vi "Inj_Array_Split.vi"(10 "Inject_Arrays":dbl[](array[numeric]), 11 "Omicron":bool) -> (0 "Air Add":dbl[](array[numeric]), 1 "Air Cyc":dbl[](array[numeric]), 2 "HC Add":dbl[](array[numeric]), 3 "HC Cyc":dbl[](array[numeric]), 4 "O2":dbl[](array[numeric]), 5 "CO":dbl[](array[numeric]), 6 "NO":dbl[](array[numeric]), 9 "Cycle Length":i32)   [LabVIEW 2014]
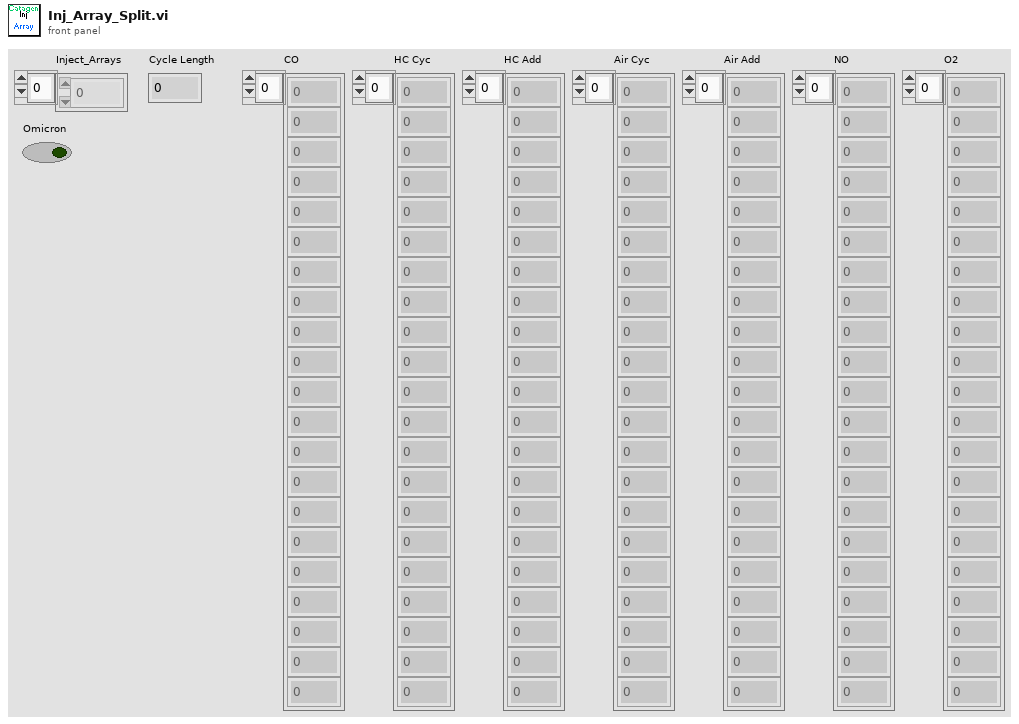
[diagram p1: front panel]
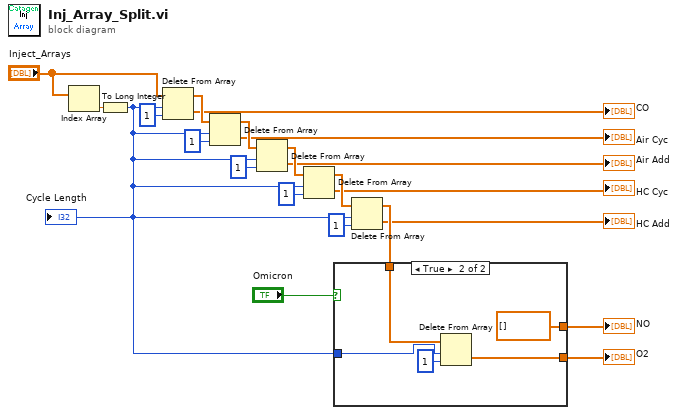
[diagram p0: block diagram]
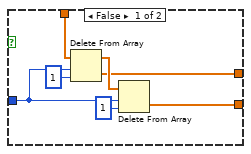
[diagram p2: hidden frame]
diagram:
  n1 = Index Array(array="Inject_Arrays") -> (element=w20:dbl)  [unwired: 1 in]
  n2 = To Long Integer(number=w20) -> (32bit integer=w2:i32)
  "Cycle Length" <- w2
  n3 = Delete From Array(array="Inject_Arrays", length=w2, index=1) -> (deleted portion=→"CO":dbl[], array with subset deleted=w19:dbl[])
  n4 = Delete From Array(array=w19, length=w2, index=1) -> (deleted portion=→"Air Cyc":dbl[], array with subset deleted=w18:dbl[])
  n5 = Delete From Array(array=w18, length=w2, index=1) -> (deleted portion=→"Air Add":dbl[], array with subset deleted=w15:dbl[])
  n6 = Delete From Array(array=w15, length=w2, index=1) -> (deleted portion=→"HC Cyc":dbl[], array with subset deleted=w13:dbl[])
  n7 = Delete From Array(array=w13, length=w2, index=1) -> (deleted portion=→"HC Add":dbl[], array with subset deleted=w10:dbl[])
  n8 = case shown="True" "Omicron" {
    tunnel: w10 -> [w25 w31]
    tunnel: [w24 dbl[] [] ("Inject_Arrays")] -> w4
    tunnel: [w23 w32] -> w3
    tunnel: w2 -> [w22 w30]
    frame False {
      n9 = Delete From Array(array=w25, length=w22, index=1) -> (deleted portion=w24:dbl[], array with subset deleted=w27:dbl[])
      n10 = Delete From Array(array=w27, length=w22, index=1) -> (deleted portion=w23:dbl[])  [unwired: 1 out]
    }
    frame True {
      n11 = Delete From Array(array=w31, length=w30, index=1) -> (deleted portion=w32:dbl[])  [unwired: 1 out]
    }
  }
  "NO" <- w4
  "O2" <- w3
